vi "CTL_SimLevelSensor.vi"(5 "Drain IN":bool, 7 "Fill IN":bool, 9 "Level PV in":dbl, 10 "Max Fill Rate":dbl=0.025, 11 "Flow Rate %":dbl=100.0) -> (3 "PV Level Inch":dbl)   [LabVIEW 2024]
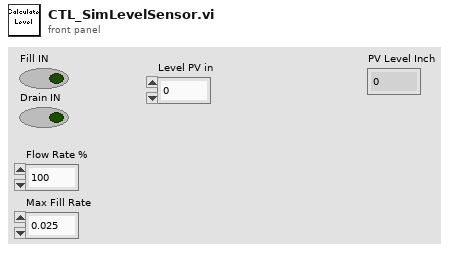
[diagram p1: front panel]
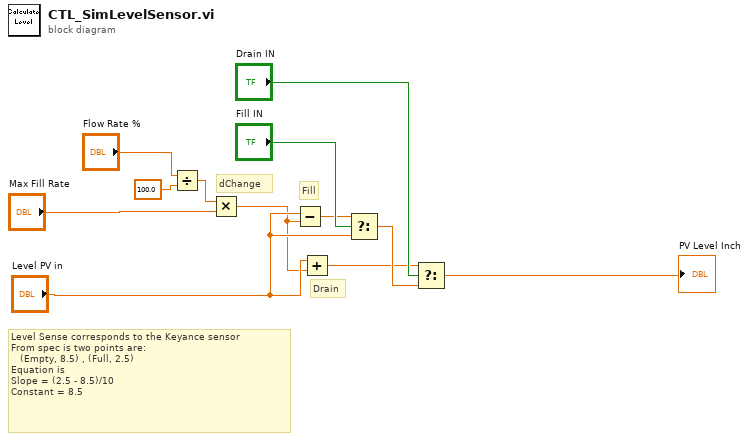
[diagram p0: block diagram]
diagram:
  # "Level Sense corresponds to the Keyance sensor\nFrom spec is two points are:\n   (Empty, 8.5) , (Full, 2.5)\nEquation is \nSlope = (2.5 - 8.5)/10\nConstant = 8.5"
  # "dChange"
  # "Drain"
  # "Fill"
  n1 = Divide(x="Flow Rate %", y=100.0) -> (x/y=w7:dbl)
  n2 = Multiply(x=w7, y="Max Fill Rate") -> (x*y=w1:dbl)
  n3 = Subtract(x="Level PV in", y=w1) -> (x-y=w3:dbl)
  n4 = Add(x="Level PV in", y=w1) -> (x+y=w4:dbl)
  n5 = Select(t=w3, s="Fill IN", f="Level PV in") -> (s? t:f=w5:dbl)
  n6 = Select(t=w4, s="Drain IN", f=w5) -> (s? t:f=→"PV Level Inch":dbl)
